vi "Simple Reader.vi"(8 "error in (no error)":errorcluster, 11 "LakeShore 370 Driver in":refnum<class "LakeShore 370 Driver.lvclass">) -> (0 "error out":errorcluster, 2 "Signals":dbl[](array[numeric]), 3 "LakeShore 370 Driver out":refnum<class "LakeShore 370 Driver.lvclass">)   [LabVIEW 2019, in "LakeShore 370 Driver.lvclass"]
uses:
  LakeShore 370 Driver.lvclass
  C:/GitHub/NHMFL_Core/Libraries/Instruments/VISA Instrument/VISA Instrument.lvclass
  VISA Instrument/VISA Instrument.lvclass/VISA Instrument.ctl
  VISA Instrument/Read VISA resource.vi
  VISA Instrument/Write VISA resource.vi
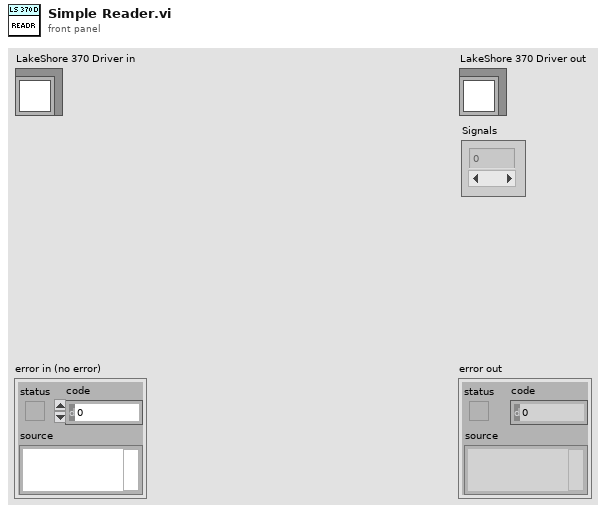
[diagram p1: front panel]
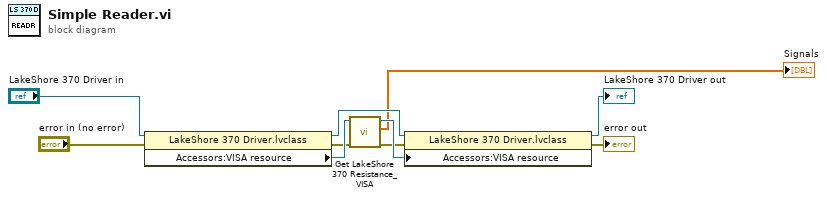
[diagram p0: block diagram]
diagram:
  n1 = property class="LakeShore 370 Driver.lvclass"(reference="LakeShore 370 Driver in", error in="error in (no error)") -> (reference out=w10:refnum<class "LakeShore 370 Driver.lvclass">, error out=w4:errorcluster, "Accessors:VISA resource"=w5:refnum<visa-resource-name>)
  n2 = call "Get LakeShore 370 Resistance_VISA.vi"("error in (no error)"=w4, "VISA resource name"=w5) -> ("error out"=w2:errorcluster, "Resistance"=→"Signals":dbl[], "VISA resource name out"=w3:refnum<visa-resource-name>)  [unwired: 7 in]
  n3 = property class="LakeShore 370 Driver.lvclass"(reference=w10, error in=w2, "Accessors:VISA resource"=w3) -> (reference out=→"LakeShore 370 Driver out":refnum<class "LakeShore 370 Driver.lvclass">, error out=→"error out":errorcluster)
